vi "Do Request.vi"(7 "Inputs":T2, 8 "error in (no error)":errorcluster, 11 "QueryAuthController in":refnum<class "QueryAuthController.lvclass">) -> (0 "error out":errorcluster, 5 "Outputs":T1)   [LabVIEW 2020, in "QueryAuthController.lvclass"]
uses:
  QueryAuthController.lvclass
  HTTP Server/Controller Inputs.ctl
  HTTP Server/Values/Values.lvclass
  <vilib>/IlluminatedG/IG HTTP Utils/HTTP Utils/Request/Request.lvclass
  HTTP Server/Session/Session.lvclass
  HTTP Server/Controller Outputs.ctl
  <vilib>/IlluminatedG/IG HTTP Utils/HTTP Utils/Response/Response.lvclass
  b94d1031-b806-4199-8881-39951c6518a9.vi
  HTTP Server/Values/Get Arg Map.vi
  <vilib>/Utility/error.llb/Error Cluster From Error Code.vi
  QueryAuthController.lvclass/QueryAuthController.ctl
  <vilib>/IlluminatedG/lv-stream/URI/URI.lvclass
  HTTP Server/HTTP Server.lvlib
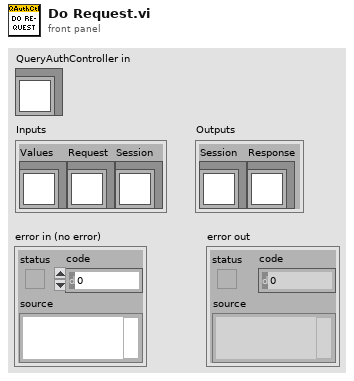
[diagram p1: front panel]
types:
  T1 = typedef "HTTP Server.lvlib/Controller Outputs.ctl" = cluster{"Session":refnum<class "Session.lvclass">, "Response":refnum<class "Response.lvclass">}
  T2 = typedef "HTTP Server.lvlib/Controller Inputs.ctl" = cluster{"Values":refnum<class "Values.lvclass">, "Request":refnum<class "Request.lvclass">, "Session":refnum<class "Session.lvclass">}
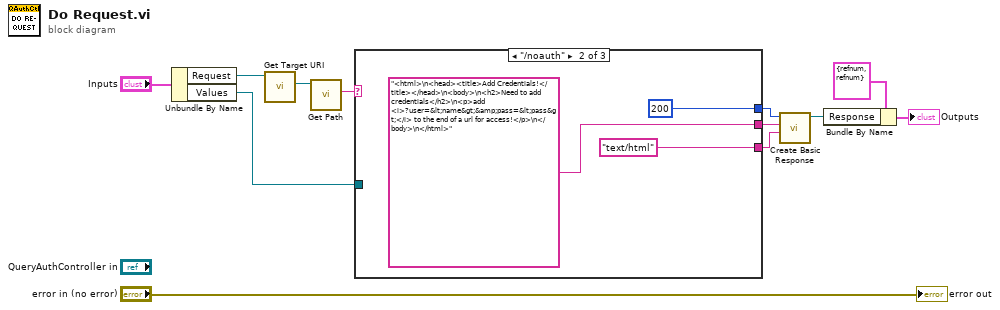
[diagram p0: block diagram]
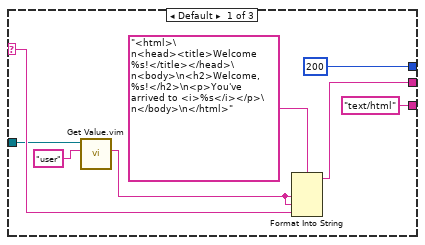
[diagram p2: hidden frame]
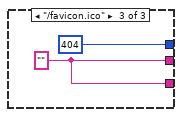
[diagram p3: hidden frame]
diagram:
  n1 = Unbundle By Name("Inputs") -> ("Request"=w5:refnum<class "Request.lvclass">, "Values"=w4:refnum<class "Values.lvclass">)
  n2 = call <vilib>:"Get Target URI.vi"("Request in"=w5) -> ("Target URI"=w11:refnum<class "URI.lvclass">)  [unwired: 8 in, 2 out]
  n3 = call <vilib>:"Get Path.vi"("URI in"=w11) -> ("Path"=w10:string)  [unwired: 8 in, 2 out]
  n4 = case shown="\"/noauth\"" w10 {
    selector: w10 -> [w16 _ _]
    tunnel: [w20 "<html>\n<head><title>Add Credentials!</title></head>\n<body>\n<h2>Need to add credentials</h2>\n<p>add <i>?user=&lt;name&gt;&amp;pass=&lt;pass&gt;</i> to the end of a url for access!</p>\n</body>\n</html>" w24] -> w8
    tunnel: [u16 200 ("Status Code") u16 200 ("Status Code") u16 404 ("Status Code")] -> w9
    tunnel: ["text/html" "text/html" w24] -> w7
    tunnel: w4 -> [w13 _ _]
    frame Default {
      n5 = call "Get Value.vim"("Name for Type"="user" ("Name for Type (Service)"), "Arguments in"=w13) -> ("Value"=w17:string)  [unwired: 7 in, 2 out]
      n6 = Format Into String(format string="<html>\n<head><title>Welcome %s!</title></head>\n<body>\n<h2>Welcome, %s!</h2>\n<p>You've arrived to <i>%s</i></p>\n</body>\n</html>", w17, w17, w16) -> (resulting string=w20:string)  [unwired: 2 in, 1 out]
    }
    frame "/noauth" {
    }
    frame "/favicon.ico" {
      w24 = ""
    }
  }
  n7 = call <vilib>:"Create Basic Response.vi"("Content-Type (text/plain)"=w7, "Payload"=w8, "Status Code"=w9) -> ("Response out"=w1:refnum<class "Response.lvclass">)  [unwired: 7 in, 1 out]
  n8 = Bundle By Name(cluster=T1 {"Session"=refnum, "Response"=refnum} ("Outputs"), "Response"=w1) -> (→"Outputs":T1)
  "error out" <- "error in (no error)"
